vi "XML Script - Function (Style String).vi"(0 "x":i32=-1, 1 "y":i32=-1, 2 "out":i32=-1, 4 "Function Style":string, 6 "name":string, 9 "prefix (name)":string, 10 "in":i32=-1) -> (5 "name (wire source)":string, 7 "XML Script Command - Function":string)   [LabVIEW 2020]
uses:
  <vilib>/_script/XML Scripting/XML Script Attribute.ctl
  <vilib>/_script/XML Scripting/XML Script Tag.ctl
panel:
  # "position"
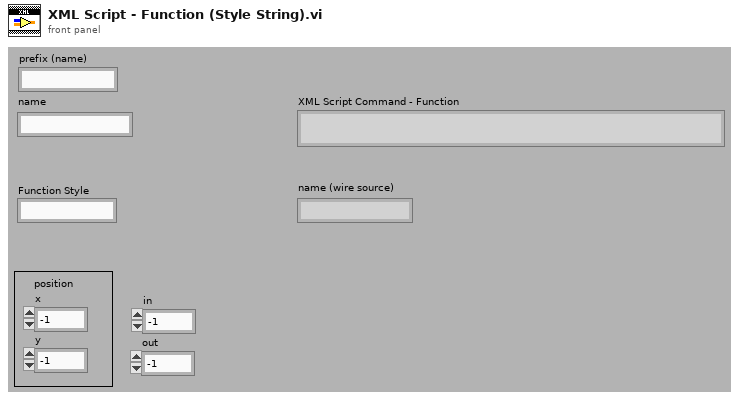
[diagram p1: front panel]
types:
  T1 = typedef "XML Script Attribute.ctl" = enum16{"name", "style", "path", "position", "in", "out", "width", "height", "index", "value", "default", "location", "offset", "typeindex", "size", "source", "destination", "indicator", "type", "controlname", "label", "conpaneidx", "mode", "description", "hasCondTerm", "linkIdentity", "caseselectortype", "concatInputs", "inName", "instantiationpath", "loopCondition", "IndexMode", "formulaInputs", "formulaOutputs", "msnFuncName", "msnIsDynamic", "msnIsODEUserFunction", "ignoreSearchDialog"}
  T2 = typedef "XML Script Tag.ctl" = enum16{"Script", "Function", "SubVI", "GrowableFunction", "Structure", "MultiframeStructure", "Frame", "Tunnel", "ShiftRegister", "Constant", "Control", "Terminal", "Wire", "StaticVIReference", "ControlTerminal", "CompoundArithmetic", "FlatSequence", "FlatSequenceFrame", "MathScriptCallByRef", "BuildArray", "GenericSubVI", "MathScriptNode"}
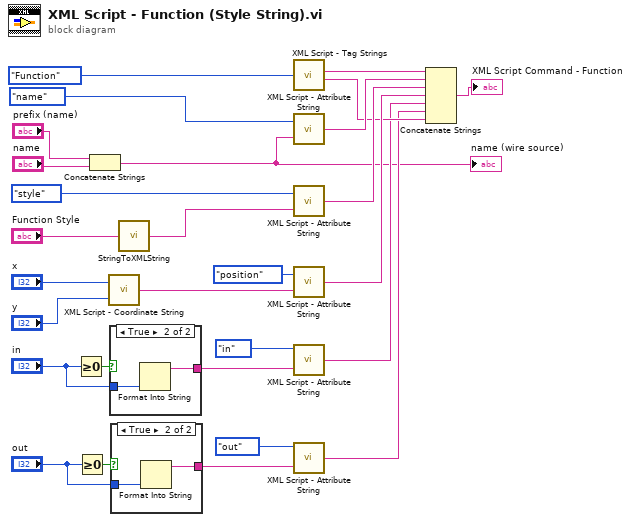
[diagram p0: block diagram]
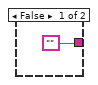
[diagram p2: hidden frame]
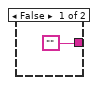
[diagram p3: hidden frame]
diagram:
  n1 = Greater Or Equal To 0?(x="in") -> (x >= 0?=w9:bool)
  n2 = Greater Or Equal To 0?(x="out") -> (x >= 0?=w13:bool)
  n3 = Concatenate Strings("prefix (name)", "name") -> (w5:string)
  "name (wire source)" <- w5
  n4 = call <vilib>:"XML Script - Coordinate String.vi"("y"="y", "x"="x") -> ("(x,y)"=w25:string)
  n5 = case shown="True" w9 {
    tunnel: "in" -> [_ w31]
    tunnel: ["" w30] -> w11
    frame False {
    }
    frame True {
      n6 = Format Into String(w31) -> (resulting string=w30:string)  [unwired: 3 in, 1 out]
    }
  }
  n7 = case shown="True" w13 {
    tunnel: "out" -> [_ w34]
    tunnel: ["" w33] -> w15
    frame False {
    }
    frame True {
      n8 = Format Into String(w34) -> (resulting string=w33:string)  [unwired: 3 in, 1 out]
    }
  }
  n9 = call <vilib>:"StringToXMLString.vi"("String"="Function Style") -> ("Valid XML String (out)"=w1:string)
  n10 = call <vilib>:"XML Script - Tag Strings.vi"("XML Script Tag"=XML_Script_Tag."Function") -> ("XML String - Begin Tag"=w22:string, "XML String - End Tag"=w16:string)  [unwired: 2 in]
  n11 = call <vilib>:"XML Script - Attribute String.vi"("Attribute String"=w5, "XML Script Attribute"=XML_Script_Attribute."name") -> ("XML Script - Attribute String"=w20:string)
  n12 = call <vilib>:"XML Script - Attribute String.vi"("Attribute String"=w1, "XML Script Attribute"=XML_Script_Attribute."style") -> ("XML Script - Attribute String"=w18:string)
  n13 = call <vilib>:"XML Script - Attribute String.vi"("Attribute String"=w25, "XML Script Attribute"=XML_Script_Attribute."position") -> ("XML Script - Attribute String"=w17:string)
  n14 = call <vilib>:"XML Script - Attribute String.vi"("Attribute String"=w11, "XML Script Attribute"=XML_Script_Attribute."in") -> ("XML Script - Attribute String"=w7:string)
  n15 = call <vilib>:"XML Script - Attribute String.vi"("Attribute String"=w15, "XML Script Attribute"=XML_Script_Attribute."out") -> ("XML Script - Attribute String"=w6:string)
  n16 = Concatenate Strings(w22, w20, w18, w17, w7, w6, w16) -> (→"XML Script Command - Function":string)
